vi "Teleop.vi"(10 "Match Info":T1={"Autonomous Elapsed Seconds"=0.0, "TeleOp Elapsed Seconds"=0.0, "Disabled Elapsed Seconds"=0.0, "Visited Autonomous"=FALSE, "Visited TeleOp"=FALSE, "Visited Disabled"=FALSE, "Autonomous Settings"={"Autonomous Style"=enum."Independent", "VI Refnum"=refnum}}, 11 "Call Context":T2) -> ()   [LabVIEW 2020]
doc: "This VI is called for each TeleOp packet received from the DS where the robot is not disabled. It is often used to read from the joysticks and update I/O or to update setpoints for timed control loops. It should complete and return within 20 milliseconds or it may miss DS packets."
uses:
  <vilib>/Rock Robotics/WPI/DriverStation/WPI_DriverStationDerivedRobotMode.ctl
  <vilib>/Rock Robotics/WPI/DriverStation/WPI_DriverStationMatch Info.ctl
  <vilib>/Rock Robotics/WPI/Utilities/WPI_GetSetVariantRefNum.vi
  <vilib>/Rock Robotics/WPI/ThirdParty/REV Robotics/REVLib/Typedef/Spark MAX Control Type.ctl
  <vilib>/Rock Robotics/WPI/ThirdParty/Phoenix-LabVIEW/CANCoder/Get/CTRE_Phoenix_CANcoder_GetSensorData.vi
panel:
  out "Yaw Graph":dbl(graph)
  # "Look inside the code for a fun suprise!"
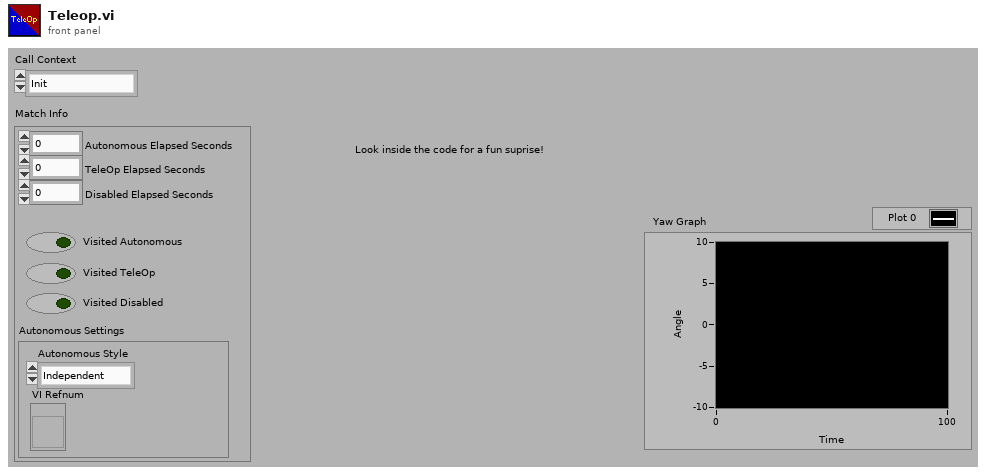
[diagram p1: front panel]
types:
  T1 = typedef "WPI_DriverStationMatch Info.ctl" = cluster{"Autonomous Elapsed Seconds":dbl, "TeleOp Elapsed Seconds":dbl, "Disabled Elapsed Seconds":dbl, "Visited Autonomous":bool, "Visited TeleOp":bool, "Visited Disabled":bool, "Autonomous Settings":cluster{"Autonomous Style":enum16{"Iterative", "Independent"}, "VI Refnum":refnum<vi>}}
  T2 = typedef "WPI_DriverStationDerivedRobotMode.ctl" = enum16{"Init", "Execute", "Stop"}
  T3 = typedef "Spark MAX Control Type.ctl" = enum16{"Percent VBus", "Voltage", "Velocity", "Position", "Smart Motion", "Current", "Smart Velocity"}
  T4 = typedef "WPI_JoystickDevRef.ctl" = cluster{"Device":T5}
  T5 = typedef "WPI_JoystickDeviceEnum.ctl" = enum16{"USB 0", "USB 1", "USB 2", "USB 3", "USB 4", "USB 5"}
  T6 = cluster{"Yaw":dbl, "Roll":dbl, "Pitch":dbl, "Heading":dbl, "Fused Heading":dbl}
  T7 = typedef "WPI_MotorControlDeviceRef.ctl" = cluster{"DeviceStatus":errorcluster, "Type":T8, "PWM":cluster{"PWM Channel":T9, "DeadBand":T10}, "CAN":cluster{"Device Number":u8, "SetOutput VI Ref":variant, "GetOutput VI Ref":variant, "Enable VI Ref":variant, "Disable VI Ref":variant, "Data":variant}, "Invert":bool, "DIO PWM":cluster{"PWM \"Enable\" Channel":T9, "DIOChannel":T11, "PWM Rate":dbl}}
  T8 = typedef "WPI_MotorControlType.ctl" = enum16{"PWM", "CAN", "DIO PWM"}
  T9 = typedef "FPGA_DIOPWMChannel.ctl" = enum8{"PWM 0", "PWM 1", "PWM 2", "PWM 3", "PWM 4", "PWM 5", "PWM 6", "PWM 7", "PWM 8", "PWM 9", "PWM MXP 0", "PWM MXP 1", "PWM MXP 2", "PWM MXP 3", "PWM MXP 4", "PWM MXP 5", "PWM MXP 6", "PWM MXP 7", "PWM MXP 8", "PWM MXP 9", "Invalid"}
  T10 = typedef "WPI_PWMDeadband.ctl" = cluster{"Name":string, "maxPositivePwm":i32, "minPositivePwm":i32, "centerPwm":i32, "maxNegativePwm":i32, "minNegativePwm":i32, "angularRange":u16}
  T11 = typedef "FPGA_DIOChannel.ctl" = enum8{"DIO 0", "DIO 1", "DIO 2", "DIO 3", "DIO 4", "DIO 5", "DIO 6", "DIO 7", "DIO 8", "DIO 9", "DIO MXP 0", "DIO MXP 1", "DIO MXP 2", "DIO MXP 3", "DIO MXP 4", "DIO MXP 5", "DIO MXP 6", "DIO MXP 7", "DIO MXP 8", "DIO MXP 9", "DIO MXP 10", "DIO MXP 11", "DIO MXP 12", "DIO MXP 13", "DIO MXP 14", "DIO MXP 15", "SPI Port CS1", "SPI Port CS2", "SPI Port CS3", "SPI Port MISO", "SPI Port MOSI", "Invalid"}
  T12 = cluster{"error out":errorcluster, "error out":errorcluster, "error out":errorcluster, "error out":errorcluster}
  T13 = cluster{"MotorControlDevRef":T7, "MotorControlDevRef":T7, "MotorControlDevRef":T7, "MotorControlDevRef":T7}
  T14 = cluster{cluster{"MotorControlDevRef":T7, "MotorControlDevRef":T7, "MotorControlDevRef":T7, "MotorControlDevRef":T7}, cluster{"error out":errorcluster, "error out":errorcluster, "error out":errorcluster, "error out":errorcluster}}
  T15 = typedef "CTRE_Phoenix_CANcoder_DeviceRef.ctl" = cluster{"DeviceStatus":errorcluster, "Device Number":u8, "Handle":u64, "UsageFrame":u32, "Library Path":path}
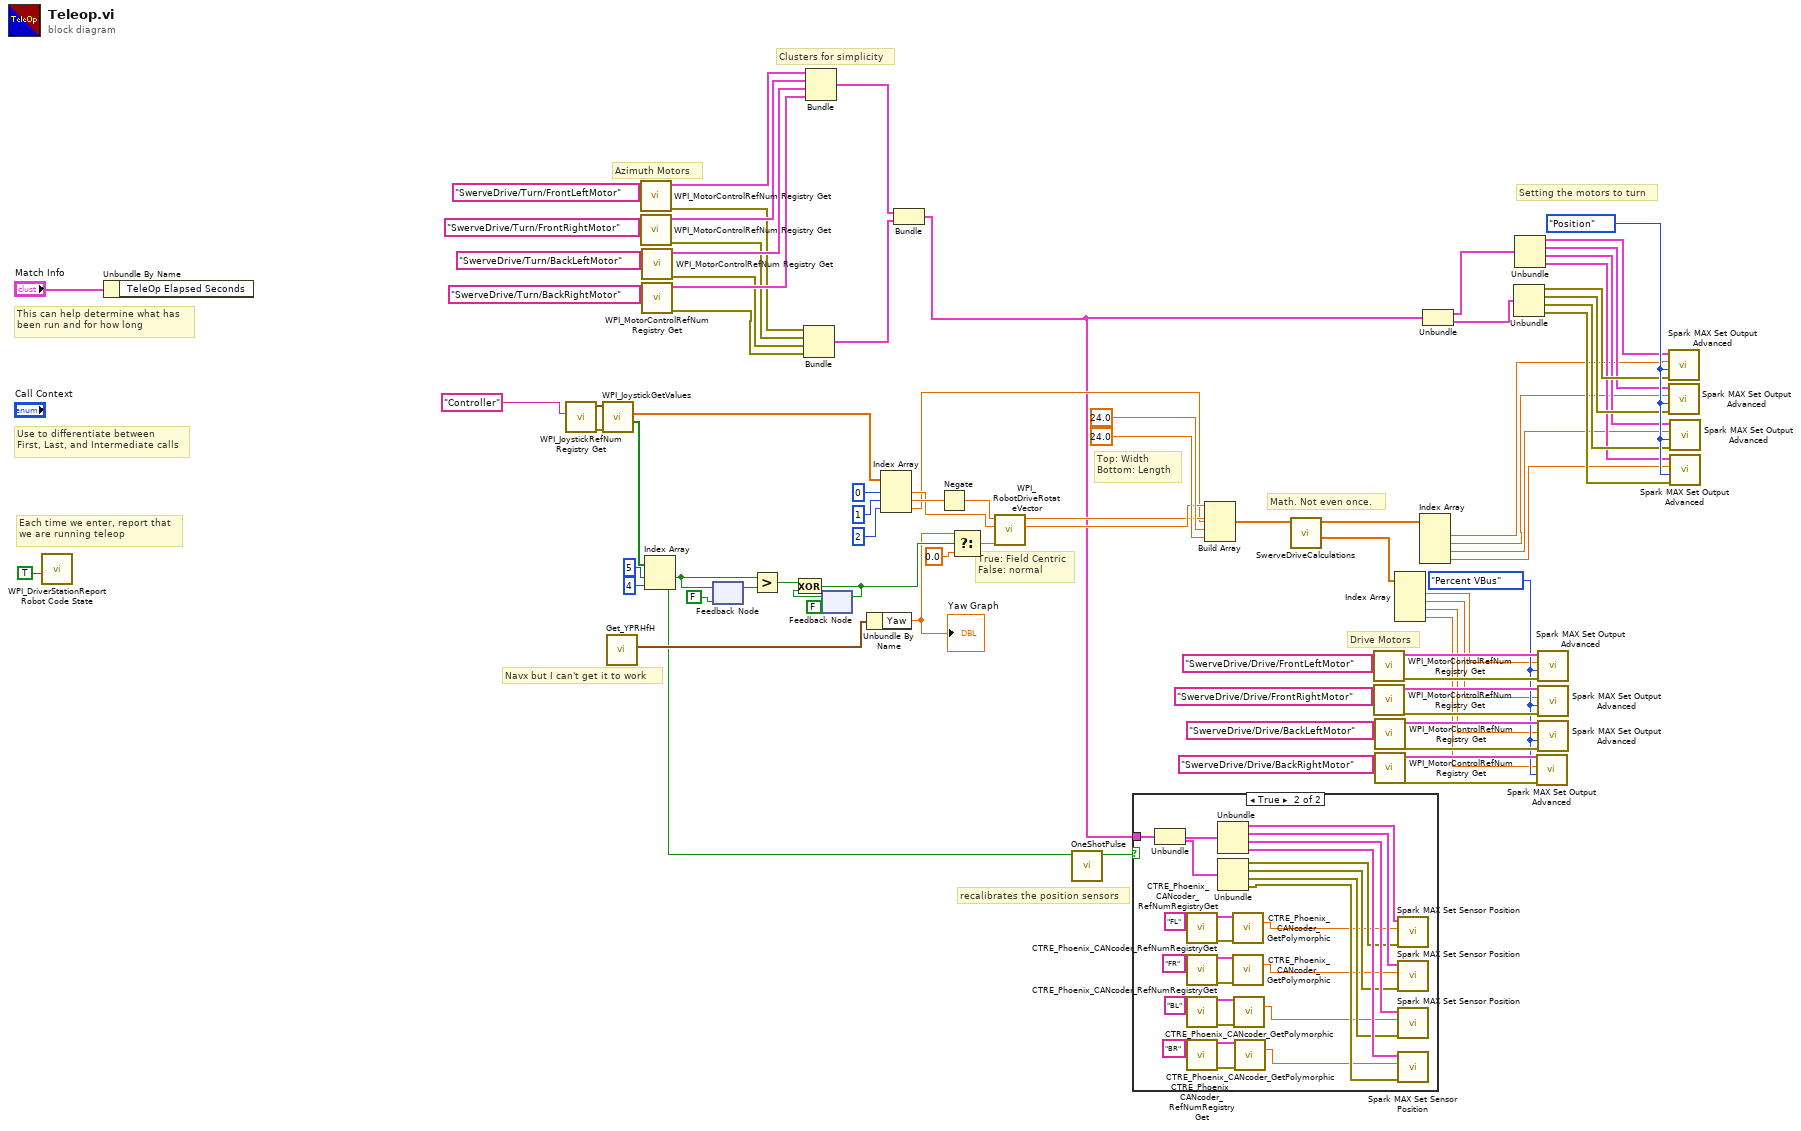
[diagram p0: block diagram]
diagram:
  w19 = Spark_MAX_Control_Type."Position" ("Control Mode")
  w44 = Spark_MAX_Control_Type."Percent VBus" ("Control Mode")
  # "Navx but I can't get it to work"
  # "Clusters for simplicity"
  # "Setting the motors to turn"
  # "Azimuth Motors"
  # "Drive Motors"
  # "recalibrates the position sensors"
  # "Math. Not even once."
  # "Top: Width\nBottom: Length"
  # "True: Field Centric\nFalse: normal"
  # "Each time we enter, report that\nwe are running teleop"
  # "Use to differentiate between\nFirst, Last, and Intermediate calls"
  # "This can help determine what has\nbeen run and for how long"
  n1 = call <vilib>:"WPI_DriverStationReport Robot Code State.vi"("TeleOp"=TRUE ("Autonomous")) -> ()  [unwired: 10 in, 1 out]
  n2 = Unbundle By Name("Match Info") -> ()  [unwired: 1 out]
  n3 = call <vilib>:"WPI_JoystickRefNum Registry Get.vi"("refnum name"="Controller") -> ("error out"=w80:errorcluster, "JoystickDevRef"=w79:T4)  [unwired: 9 in]
  n4 = call <vilib>:"WPI_JoystickGetValues.vi"("error in (no error)"=w80, "JoystickDevRef"=w79) -> ("Buttons"=w78:bool[], "Axes"=w77:dbl[])  [unwired: 5 in, 3 out]
  n5 = call <vilib>:"Get_YPRHfH.vi"() -> ("YRPHfH"=w69:T6)  [unwired: 11 in]
  n6 = call <vilib>:"WPI_MotorControlRefNum Registry Get.vi"("refnum name"="SwerveDrive/Turn/FrontLeftMotor") -> ("error out"=w25:errorcluster, "MotorControlDevRef"=w26:T7)  [unwired: 9 in]
  n7 = call <vilib>:"WPI_MotorControlRefNum Registry Get.vi"("refnum name"="SwerveDrive/Turn/FrontRightMotor") -> ("error out"=w24:errorcluster, "MotorControlDevRef"=w27:T7)  [unwired: 9 in]
  n8 = call <vilib>:"WPI_MotorControlRefNum Registry Get.vi"("refnum name"="SwerveDrive/Turn/BackLeftMotor") -> ("error out"=w23:errorcluster, "MotorControlDevRef"=w28:T7)  [unwired: 9 in]
  n9 = call <vilib>:"WPI_MotorControlRefNum Registry Get.vi"("refnum name"="SwerveDrive/Turn/BackRightMotor") -> ("error out"=w22:errorcluster, "MotorControlDevRef"=w29:T7)  [unwired: 9 in]
  n10 = Index Array(array=w78, index #1=5 ("index"), index #2=4 ("index")) -> (element #1=w66:bool, element #2=w5:bool)
  n11 = feedback #1(FALSE) -> (w67:bool)
  n12 = feedback-in #1(w66) -> ()
  n13 = Greater?(x=w66, y=w67) -> (0:w65:bool)
  n14 = Bundle("error out"=w25, "error out"=w24, "error out"=w23, "error out"=w22) -> (w20:T12)  [unwired: 1 in]
  n15 = Bundle("MotorControlDevRef"=w26, "MotorControlDevRef"=w27, "MotorControlDevRef"=w28, "MotorControlDevRef"=w29) -> (w21:T13)  [unwired: 1 in]
  n16 = feedback #2(FALSE) -> (w64:bool)
  n17 = Exclusive Or(1:w64, 2:w65) -> (0:w62:bool)
  n18 = feedback-in #2(w62) -> ()
  n19 = Unbundle By Name(w69) -> ("Yaw"=w61:dbl)
  "Yaw Graph" <- w61
  n20 = Index Array(array=w77, index #1=0 ("index"), index #2=1 ("index"), index #3=2 ("index")) -> (element #1=w70:dbl, element #2=w72:dbl, element #3=w54:dbl)
  n21 = Bundle(w21, w20) -> (w7:T14)  [unwired: 1 in]
  n22 = Negate(x=w72) -> (-x=w71:dbl)
  n23 = Select(t=w61, s=w62, f=0.0) -> (s? t:f=w59:dbl)
  n24 = call <vilib>:"WPI_RobotDriveRotateVector.vi"("Angle"=w59, "X"=w70, "Y"=w71) -> ("X'"=w56:dbl, "Y'"=w55:dbl)  [unwired: 7 out]
  n25 = call "OneShotPulse.vi"("Input"=w5) -> ("Output"=w6:bool)  [unwired: 10 in]
  n26 = case shown="True" w6 {
    tunnel: w7 -> [_ w110]
    frame False {
    }
    frame True {
      n27 = Unbundle(w110) -> (w109:T13, w108:T12)
      n28 = call <vilib>:"CTRE_Phoenix_CANcoder_RefNumRegistryGet.vi"("refnum name"="FL") -> ("error out"=w98:errorcluster, "CTRE_CANcoder_DeviceRef"=w99:T15)  [unwired: 9 in]
      n29 = call <vilib>:"CTRE_Phoenix_CANcoder_RefNumRegistryGet.vi"("refnum name"="FR") -> ("error out"=w96:errorcluster, "CTRE_CANcoder_DeviceRef"=w97:T15)  [unwired: 9 in]
      n30 = call <vilib>:"CTRE_Phoenix_CANcoder_RefNumRegistryGet.vi"("refnum name"="BL") -> ("error out"=w94:errorcluster, "CTRE_CANcoder_DeviceRef"=w95:T15)  [unwired: 9 in]
      n31 = call <vilib>:"CTRE_Phoenix_CANcoder_RefNumRegistryGet.vi"("refnum name"="BR") -> ("error out"=w92:errorcluster, "CTRE_CANcoder_DeviceRef"=w93:T15)  [unwired: 9 in]
      n32 = Unbundle(w109) -> ("MotorControlDevRef"=w107:T7, "MotorControlDevRef"=w106:T7, "MotorControlDevRef"=w105:T7, "MotorControlDevRef"=w104:T7)
      n33 = Unbundle(w108) -> ("error out"=w103:errorcluster, "error out"=w102:errorcluster, "error out"=w101:errorcluster, "error out"=w100:errorcluster)
      n34 = call-poly <vilib>:"CTRE_Phoenix_CANcoder_GetPolymorphic.vi"("CTRE_CANcoder_DeviceRef"=w99, "error in"=w98) -> ("Position"=w88:dbl)  [unwired: 9 in, 4 out]
      n35 = call-poly <vilib>:"CTRE_Phoenix_CANcoder_GetPolymorphic.vi"("CTRE_CANcoder_DeviceRef"=w97, "error in"=w96) -> ("Position"=w89:dbl)  [unwired: 9 in, 4 out]
      n36 = call-poly <vilib>:"CTRE_Phoenix_CANcoder_GetPolymorphic.vi"("CTRE_CANcoder_DeviceRef"=w95, "error in"=w94) -> ("Position"=w90:dbl)  [unwired: 9 in, 4 out]
      n37 = call-poly <vilib>:"CTRE_Phoenix_CANcoder_GetPolymorphic.vi"("CTRE_CANcoder_DeviceRef"=w93, "error in"=w92) -> ("Position"=w91:dbl)  [unwired: 9 in, 4 out]
      n38 = call <vilib>:"Spark MAX Set Sensor Position.vi"("error in"=w103, "Position"=w88, "MotorControlDeviceRef"=w107) -> ()  [unwired: 7 in, 2 out]
      n39 = call <vilib>:"Spark MAX Set Sensor Position.vi"("error in"=w102, "Position"=w89, "MotorControlDeviceRef"=w106) -> ()  [unwired: 7 in, 2 out]
      n40 = call <vilib>:"Spark MAX Set Sensor Position.vi"("error in"=w101, "Position"=w90, "MotorControlDeviceRef"=w105) -> ()  [unwired: 7 in, 2 out]
      n41 = call <vilib>:"Spark MAX Set Sensor Position.vi"("error in"=w100, "Position"=w91, "MotorControlDeviceRef"=w104) -> ()  [unwired: 7 in, 2 out]
    }
  }
  n42 = Build Array(w56, w55, w54, 24.0 ("element"), 24.0 ("element")) -> (w53:dbl[])
  n43 = call "SwerveDriveCalculations.vi"("SwerveCommands"=w53) -> ("Velocity"=w43:dbl[], "Angle"=w34:dbl[])  [unwired: 9 in]
  n44 = call <vilib>:"WPI_MotorControlRefNum Registry Get.vi"("refnum name"="SwerveDrive/Drive/FrontLeftMotor") -> ("error out"=w46:errorcluster, "MotorControlDevRef"=w45:T7)  [unwired: 9 in]
  n45 = call <vilib>:"WPI_MotorControlRefNum Registry Get.vi"("refnum name"="SwerveDrive/Drive/FrontRightMotor") -> ("error out"=w48:errorcluster, "MotorControlDevRef"=w47:T7)  [unwired: 9 in]
  n46 = call <vilib>:"WPI_MotorControlRefNum Registry Get.vi"("refnum name"="SwerveDrive/Drive/BackLeftMotor") -> ("error out"=w50:errorcluster, "MotorControlDevRef"=w49:T7)  [unwired: 9 in]
  n47 = call <vilib>:"WPI_MotorControlRefNum Registry Get.vi"("refnum name"="SwerveDrive/Drive/BackRightMotor") -> ("error out"=w51:errorcluster, "MotorControlDevRef"=w52:T7)  [unwired: 9 in]
  n48 = Index Array(array=w43) -> (element #1=w39:dbl, element #2=w40:dbl, element #3=w41:dbl, element #4=w42:dbl)  [unwired: 4 in]
  n49 = Index Array(array=w34) -> (element #1=w4:dbl, element #2=w3:dbl, element #3=w2:dbl, element #4=w1:dbl)  [unwired: 4 in]
  n50 = Unbundle(w7) -> (w18:T13, w17:T12)
  n51 = Unbundle(w17) -> ("error out"=w13:errorcluster, "error out"=w14:errorcluster, "error out"=w15:errorcluster, "error out"=w16:errorcluster)
  n52 = Unbundle(w18) -> ("MotorControlDevRef"=w9:T7, "MotorControlDevRef"=w10:T7, "MotorControlDevRef"=w11:T7, "MotorControlDevRef"=w12:T7)
  n53 = call <vilib>:"Spark MAX Set Output Advanced.vi"("error in (no error)"=w51, "Control Mode"=w44, "Setpoint"=w42, "MotorControlDevRef"=w52) -> ()  [unwired: 6 in, 2 out]
  n54 = call <vilib>:"Spark MAX Set Output Advanced.vi"("error in (no error)"=w46, "Control Mode"=w44, "Setpoint"=w39, "MotorControlDevRef"=w45) -> ()  [unwired: 6 in, 2 out]
  n55 = call <vilib>:"Spark MAX Set Output Advanced.vi"("error in (no error)"=w48, "Control Mode"=w44, "Setpoint"=w40, "MotorControlDevRef"=w47) -> ()  [unwired: 6 in, 2 out]
  n56 = call <vilib>:"Spark MAX Set Output Advanced.vi"("error in (no error)"=w50, "Control Mode"=w44, "Setpoint"=w41, "MotorControlDevRef"=w49) -> ()  [unwired: 6 in, 2 out]
  n57 = call <vilib>:"Spark MAX Set Output Advanced.vi"("error in (no error)"=w13, "Control Mode"=w19, "Setpoint"=w4, "MotorControlDevRef"=w9) -> ()  [unwired: 6 in, 2 out]
  n58 = call <vilib>:"Spark MAX Set Output Advanced.vi"("error in (no error)"=w14, "Control Mode"=w19, "Setpoint"=w3, "MotorControlDevRef"=w10) -> ()  [unwired: 6 in, 2 out]
  n59 = call <vilib>:"Spark MAX Set Output Advanced.vi"("error in (no error)"=w15, "Control Mode"=w19, "Setpoint"=w2, "MotorControlDevRef"=w11) -> ()  [unwired: 6 in, 2 out]
  n60 = call <vilib>:"Spark MAX Set Output Advanced.vi"("error in (no error)"=w16, "Control Mode"=w19, "Setpoint"=w1, "MotorControlDevRef"=w12) -> ()  [unwired: 6 in, 2 out]
